vi "SaveConfig.vi"(8 "path to XML document":path, 9 "USB/RS170 cams":bool, 10 "CamerasNames":string[](array[string]), 11 "DeviceConfigArray":T2(array[cluster]) {"CorrectConfig Cluster"."Acquisition Parameters"."White level" scale=0.3..1.26 scale format="%#_2f"; "CorrectConfig Cluster"."Acquisition Parameters"."Saturation" scale=0.5..1.5 scale format="%#_3f"; "CorrectConfig Cluster"."Acquisition Parameters"."Contrast" scale=0.4..1.5 scale format="%#_3f"; "CorrectConfig Cluster"."Acquisition Parameters"."Brightness" scale=-50.0..50.0 scale format="%#_2f"; "CorrectConfig Cluster"."Correction Parameters"."Movement Type" items=["Step", "Proportionnal"]; "CorrectConfig Cluster"."Target"."X Target" format="%#_5g"; "CorrectConfig Cluster"."Target"."Y Target" format="%#_5g"; "CorrectConfig Cluster"."Detection Parameters"."Max Intensity%" max=100 step=1}) -> (0 "error out":errorcluster)   [LabVIEW 2013]
uses:
  <vilib>/userdefined/High Color/IMAQdx.ctl
  <vilib>/xml/Load XML File.vi
  <resource>/objmgr/DOMUserDefRef.rc
  <vilib>/xml/NI_XML.lvlib
panel:
  out "parse errors":string
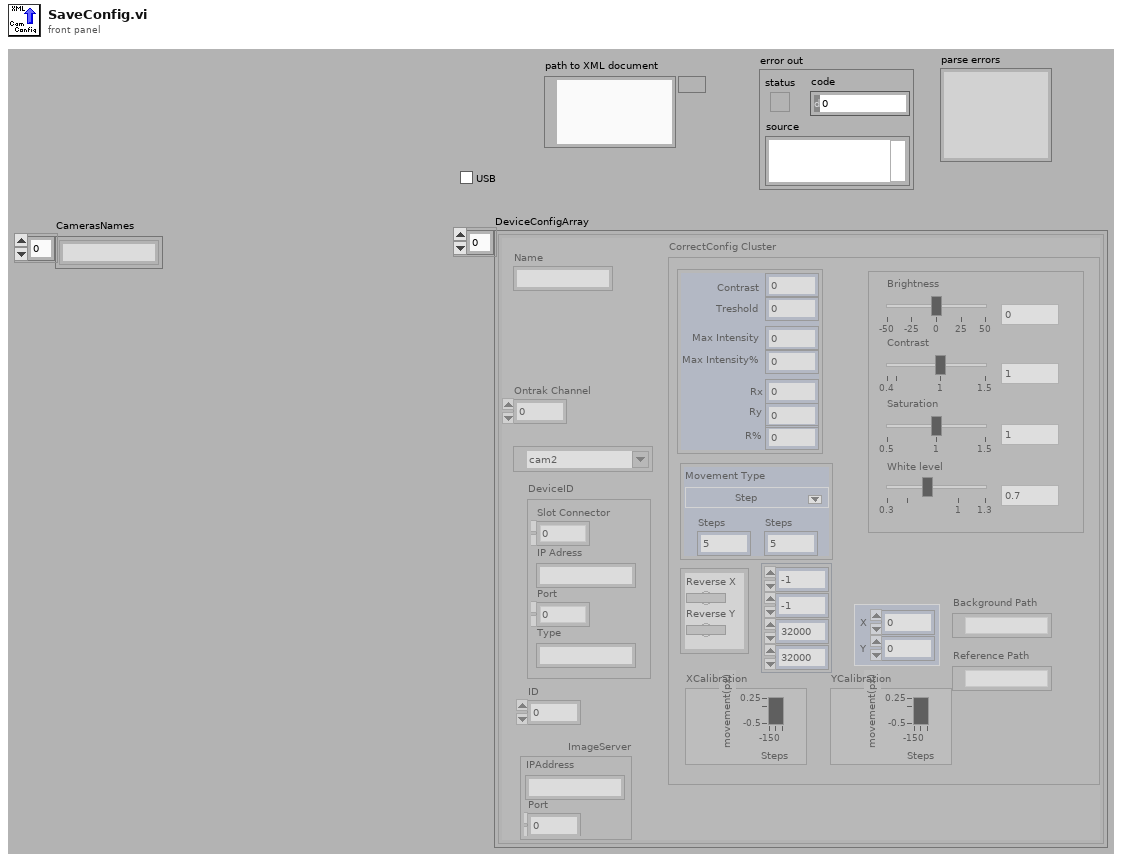
[diagram p1: front panel]
types:
  T1 = typedef "IMAQdx.ctl" = refnum<k21>
  T2 = cluster{"ID":dbl, "Name":string, "DeviceID":cluster{"Slot Connector":i32, "IP Adress":string, "Port":i32, "Type":string}, "CorrectConfig Cluster":cluster{"Detection Parameters":cluster{"Contrast":i32, "Treshold":u8, "Max Intensity":i32, "Max Intensity%":u8, "Rx":i32, "Ry":i32, "R%":sgl}, "Reverse":cluster{"Reverse X":bool, "Reverse Y":bool}, "Target":cluster{"X Target":sgl, "Y Target":sgl}, "Region of Interest":i32[], "Correction Parameters":cluster{"X":sgl, "Y":sgl, "Movement Type":u16}, "Acquisition Parameters":cluster{"Brightness":dbl, "Contrast":dbl, "Saturation":dbl, "White level":dbl}, "Background Path":path, "Reference Path":path, "XCalibration":cluster{dbl, dbl}[], "YCalibration":cluster{dbl, dbl}[]}, "Ontrak Channel":i16, "IMAQdx Session":T1, "ImageServer":cluster{"IPAddress":string, "Port":i32}}[]
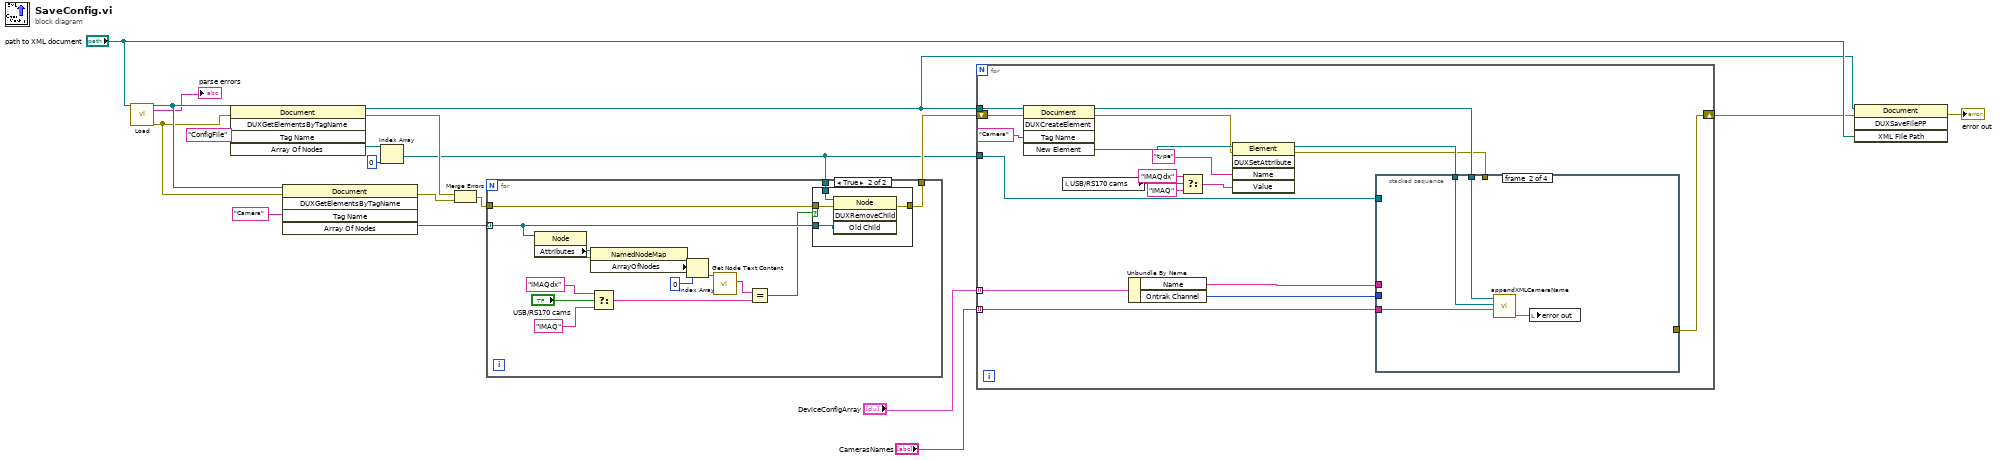
[diagram p0: block diagram]
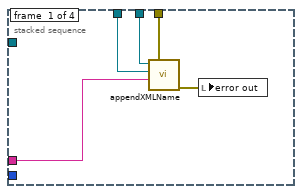
[diagram p3: hidden frame]
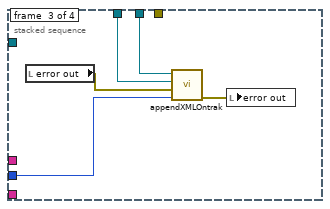
[diagram p4: hidden frame]
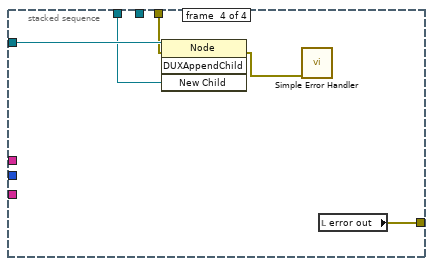
[diagram p5: hidden frame]
diagram:
  n1 = call-poly <vilib>:"Load.vi"("path to XML document"="path to XML document") -> ("DOM document out"=w16:refnum<k20>, "parse errors"=→"parse errors":string, "error out"=w14:errorcluster)  [unwired: 12 in]
  n2 = invoke class="Document" method="DUXGetElementsByTagName"(reference=w16, error in=w14, "Tag Name"="ConfigFile") -> (reference out=w1:refnum<k20>, error out=w12:errorcluster, "Array Of Nodes"=w18:refnum<k20>[])  [unwired: 2 in, 2 out]
  n3 = invoke class="Document" method="DUXGetElementsByTagName"(reference=w16, error in=w14, "Tag Name"="Camera") -> (error out=w11:errorcluster, "Array Of Nodes"=w15:refnum<k20>[])  [unwired: 2 in, 3 out]
  n4 = Index Array(array=w18, index=0) -> (element=w9:refnum<k20>)
  n5 = Merge Errors(w12, w11) -> (w13:errorcluster)
  n6 = for {
    tunnel: w9 -> [w34]
    tunnel: w15 -> [w23] mode=indexing
    tunnel: [w33] -> w10
    tunnel: w13 -> [w32]
    n7 = property class="Node"(reference=w23) -> (error out=w27:errorcluster, "Attributes"=w28:refnum<k20>)  [unwired: 1 in, 1 out]
    n8 = property class="NamedNodeMap"(reference=w28, error in=w27) -> ("ArrayOfNodes"=w26:refnum<k20>[])  [unwired: 2 out]
    n9 = Select(t="IMAQdx", s="USB/RS170 cams", f="IMAQ") -> (s? t:f=w21:string)
    n10 = Index Array(array=w26, index=0) -> (element=w24:refnum<k20>)
    n11 = call <vilib>:"Get Node Text Content.vi"("node in"=w24) -> ("node text"=w22:string)  [unwired: 8 in, 2 out]
    n12 = Equal?(x=w22, y=w21) -> (x = y?=w20:bool)
    n13 = case shown="True" w20 {
      tunnel: w34 -> [_ w39]
      tunnel: [w35 w38] -> w33
      tunnel: w32 -> [w35 w37]
      tunnel: w23 -> [_ w36]
      frame False {
      }
      frame True {
        n14 = invoke class="Node" method="DUXRemoveChild"(reference=w39, error in=w37, "Old Child"=w36) -> (error out=w38:errorcluster)  [unwired: 1 in, 3 out]
      }
    }
  }
  n15 = for {
    tunnel: "DeviceConfigArray" -> [w58] mode=indexing
    tunnel: w1 -> [w47]
    tunnel: w9 -> [w53]
    shift-right: [w52] -> w3
    shift-left: w10 -> [w54]
    tunnel: "CamerasNames" -> [w40] mode=indexing
    n16 = invoke class="Document" method="DUXCreateElement"(reference=w47, error in=w54, "Tag Name"="Camera") -> (reference out=w55:refnum<k20>, error out=w42:errorcluster, "New Element"=w44:refnum<k20>)  [unwired: 2 in, 2 out]
    n17 = local read "USB/RS170 cams"() -> (w49:bool)
    n18 = Unbundle By Name(w58) -> ("Name"=w57:string, "Ontrak Channel"=w56:i16)
    n19 = Select(t="IMAQdx" ("Tag Name"), s=w49, f="IMAQ" ("Tag Name")) -> (s? t:f=w46:string)
    n20 = invoke class="Element" method="DUXSetAttribute"(reference=w44, error in=w42, "Name"="type", "Value"=w46) -> (reference out=w43:refnum<k20>, error out=w41:errorcluster)  [unwired: 1 in, 3 out]
    n21 = stacked-sequence {
      tunnel: w43 -> [w62 w64 w71 w76]
      tunnel: w55 -> [w61 w65 w72 _]
      tunnel: w57 -> [w63 _ _ _]
      tunnel: w56 -> [_ _ w70 _]
      tunnel: w53 -> [_ _ _ w77]
      tunnel: w41 -> [w60 _ _ w75]
      tunnel: [_ _ _ w73] -> w52
      tunnel: w40 -> [_ w66 _ _]
      frame #0 {
        n22 = call "appendXMLName.vi"("error in (no error)"=w60, "name"=w63, "Parent Device Node"=w62, "DOM document in"=w61) -> ("error out"=w59:errorcluster)  [unwired: 7 in]
        n23 = local write "error out"(w59) -> ()
      }
      frame #1 {
        n24 = call "appendXMLCameraName.vi"("name"=w66, "Parent Device Node"=w64, "DOM document in"=w65) -> ("error out"=w67:errorcluster)  [unwired: 8 in]
        n25 = local write "error out"(w67) -> ()
      }
      frame #2 {
        n26 = local read "error out"() -> (w69:errorcluster)
        n27 = call "appendXMLOntrak.vi"("Ontrak Channel"=w70, "error in (no error)"=w69, "Parent Camera Node"=w71, "DOM document in"=w72) -> ("error out"=w68:errorcluster)  [unwired: 7 in]
        n28 = local write "error out"(w68) -> ()
      }
      frame #3 {
        n29 = invoke class="Node" method="DUXAppendChild"(reference=w77, error in=w75, "New Child"=w76) -> (error out=w74:errorcluster)  [unwired: 1 in, 3 out]
        n30 = call <vilib>:"Simple Error Handler.vi"("error in (no error)"=w74) -> ()  [unwired: 4 in, 5 out]
        n31 = local read "error out"() -> (w73:errorcluster)
      }
    }
  }
  n32 = invoke class="Document" method="DUXSaveFilePP"(reference=w1, error in=w3, "XML File Path"="path to XML document") -> (error out=→"error out":errorcluster)  [unwired: 1 in, 3 out]
